vi "Comparison.vi"(7 "Comparison Mode":T2, 10 "value":dbl, 11 "minMax":T1) -> (2 "result":bool)   [LabVIEW 2018]
uses:
  comparison mode.ctl
  Min_Max.ctl
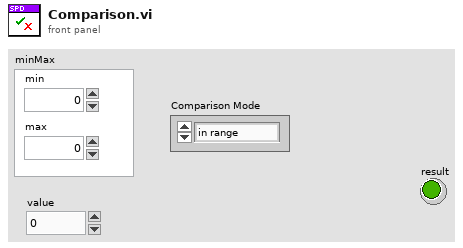
[diagram p1: front panel]
types:
  T1 = typedef "Min_Max.ctl" = cluster{"min":dbl, "max":dbl}
  T2 = typedef "comparison mode.ctl" = enum16{"in range", "bigger then min", "bigger then max", "less then min", "less then max"}
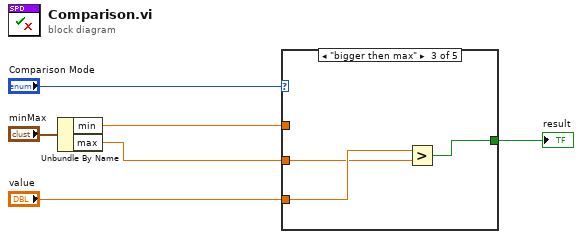
[diagram p0: block diagram]
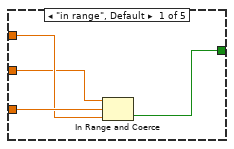
[diagram p2: hidden frame]
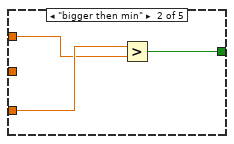
[diagram p3: hidden frame]
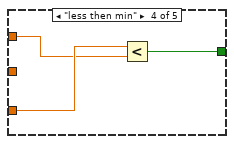
[diagram p4: hidden frame]
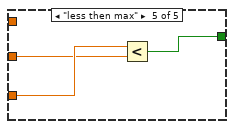
[diagram p5: hidden frame]
diagram:
  n1 = Unbundle By Name("minMax") -> ("min"=w2:dbl, "max"=w1:dbl)
  n2 = case shown="\"bigger then max\"" "Comparison Mode" {
    tunnel: w2 -> [w8 w11 _ w17 _]
    tunnel: w1 -> [w7 _ w14 _ w20]
    tunnel: "value" -> [w10 w13 w16 w19 w21]
    tunnel: [w9 w12 w15 w18 w22] -> w4
    frame "in range", Default {
      n3 = In Range and Coerce(upper limit=w7, x=w10, lower limit=w8) -> (In Range?=w9:bool)  [unwired: 1 out]
    }
    frame "bigger then min" {
      n4 = Greater?(x=w13, y=w11) -> (0:w12:bool)
    }
    frame "bigger then max" {
      n5 = Greater?(x=w16, y=w14) -> (0:w15:bool)
    }
    frame "less then min" {
      n6 = Less?(x=w19, y=w17) -> (x < y?=w18:bool)
    }
    frame "less then max" {
      n7 = Less?(x=w21, y=w20) -> (x < y?=w22:bool)
    }
  }
  "result" <- w4
